vi "Set Root Node Properties and Name.vi"(4 "Description":string, 6 "Creator":string, 7 "Skip search (F)":bool, 8 "error in (no error)":errorcluster, 9 "Name":string, 10 "guid":string, 11 "Doc in":refnum<k24>) -> (0 "error out":errorcluster, 3 "Doc out":refnum<k24>)   [LabVIEW 2013, in "Project Wizard.lvlib"]
uses:
  Project Wizard.lvlib
  NationalInstruments.VeriStand.SystemStorage
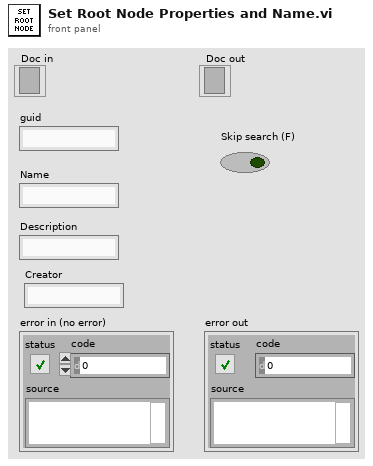
[diagram p1: front panel]
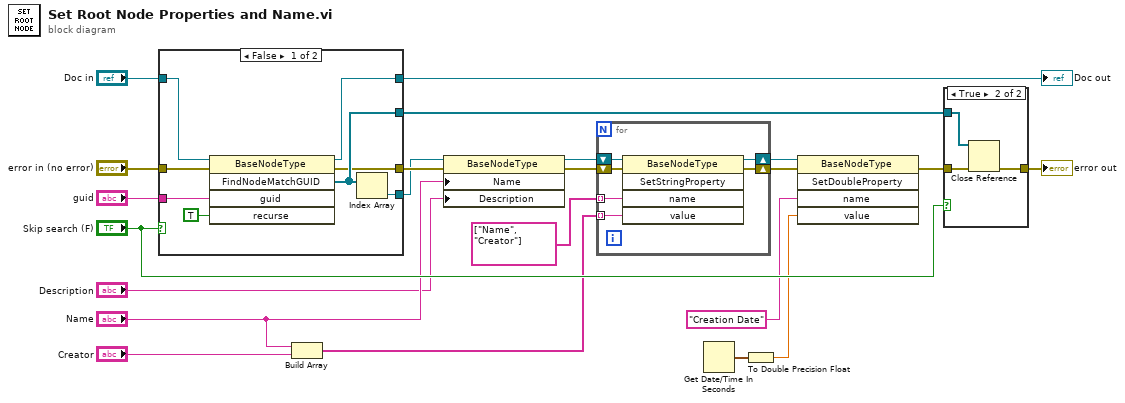
[diagram p0: block diagram]
diagram:
  n1 = case shown="False" "Skip search (F)" {
    tunnel: [w30 w31] -> w22
    tunnel: "guid" -> [w29 _]
    tunnel: "Doc in" -> [w28 w31]
    tunnel: "error in (no error)" -> [w27 w32]
    tunnel: [w26 _] -> w17
    tunnel: [w25 w32] -> w14
    tunnel: [w24 w31] -> w13
    frame False {
      n2 = invoke class="BaseNodeType" method="FindNodeMatchGUID"(reference=w28, error in=w27, "guid"=w29, "recurse"=TRUE) -> (reference out=w30:refnum<k24>, error out=w25:errorcluster, "FindNodeMatchGUID"=w26:refnum<k24>[])  [unwired: 1 in, 2 out]
      n3 = Index Array(array=w26) -> (element=w24:refnum<k24>)  [unwired: 1 in]
    }
    frame True {
    }
  }
  "Doc out" <- w22
  n4 = Build Array("Name", "Creator") -> (w8:string[])
  n5 = property class="BaseNodeType"(reference=w13, error in=w14, "Name"="Name", "Description"="Description") -> (reference out=w15:refnum<k24>, error out=w16:errorcluster)
  n6 = for {
    tunnel: w8 -> [w38] mode=indexing
    tunnel: string[] ["Name", "Creator"] -> [w37] mode=indexing
    shift-right: [w34] -> w7
    shift-left: w16 -> [w36]
    shift-right: [w33] -> w6
    shift-left: w15 -> [w35]
    n7 = invoke class="BaseNodeType" method="SetStringProperty"(reference=w35, error in=w36, "name"=w37, "value"=w38) -> (reference out=w33:refnum<k24>, error out=w34:errorcluster)  [unwired: 1 in, 3 out]
  }
  n8 = Get Date/Time In Seconds() -> (seconds since 1Jan1904=w4:timestamp)
  n9 = To Double Precision Float(number=w4) -> (double precision float=w3:dbl)
  n10 = invoke class="BaseNodeType" method="SetDoubleProperty"(reference=w6, error in=w7, "name"="Creation Date", "value"=w3) -> (error out=w2:errorcluster)  [unwired: 1 in, 4 out]
  n11 = case shown="True" "Skip search (F)" {
    tunnel: [w39 w42] -> w21
    tunnel: w17 -> [_ w41]
    tunnel: w2 -> [w39 w40]
    frame False {
    }
    frame True {
      n12 = Close Reference(reference=w41, error in (no error)=w40) -> (error out=w42:errorcluster)
    }
  }
  "error out" <- w21
